vi "Key Fob Lock Press.vi"(8 "error in (no error)":errorcluster, 11 "VehicleModelPlatinum in":refnum<class "VehicleModelPlatinum.lvclass">) -> (0 "error out":errorcluster, 1 "Report Text":string, 2 "Test Result":bool, 3 "VehicleModelPlatinum out":refnum<class "VehicleModelPlatinum.lvclass">)   [LabVIEW 2024, in "VehicleModelPlatinum.lvclass"]
uses:
  VehicleModelPlatinum.lvclass
  VehicleModelPlatinum.lvclass/VehicleModelPlatinum.ctl
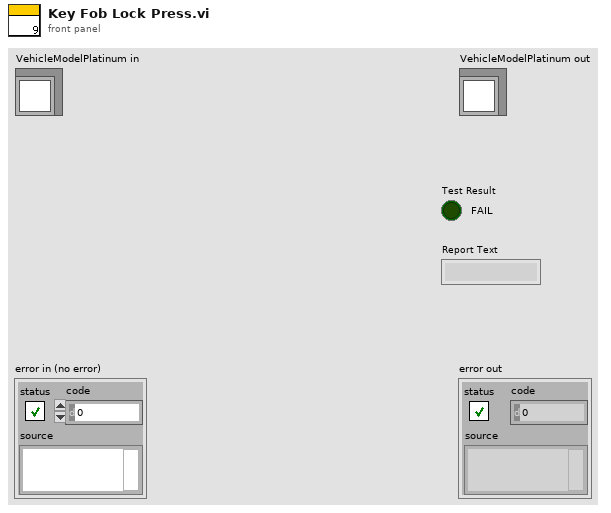
[diagram p1: front panel]
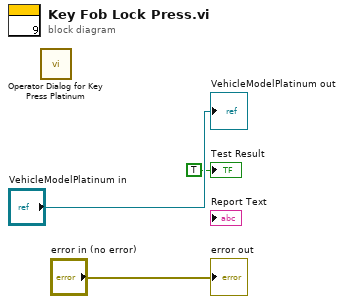
[diagram p0: block diagram]
diagram:
  n1 = call "Operator Dialog for Key Press Platinum.vi"() -> ()  [unwired: 12 in]
  "error out" <- "error in (no error)"
  "VehicleModelPlatinum out" <- "VehicleModelPlatinum in"
  "Test Result" <- TRUE ("Test Result")
